vi "HV Onstate Multi.vi"(8 "On/Off":string[](array[string]), 11 "Channel":string[](array[string])) -> (3 "standard output":string)   [LabVIEW 2018, in "HV QMH.lvlib"]
uses:
  HV QMH.lvlib
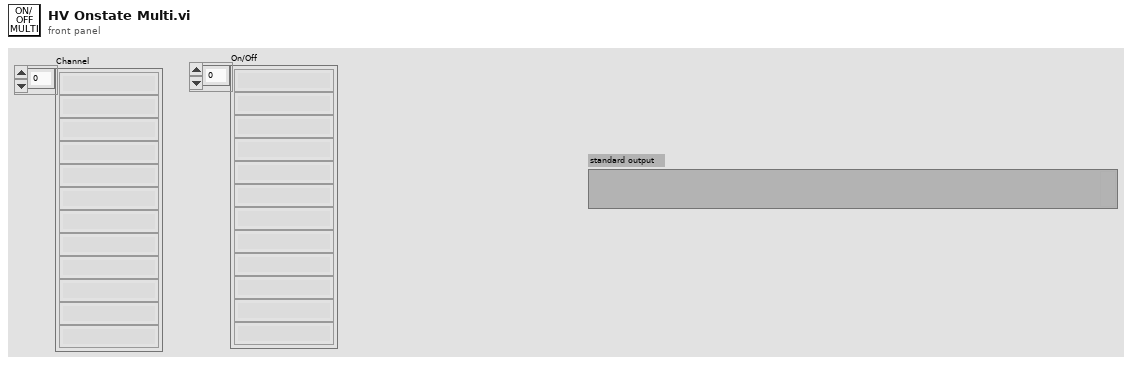
[diagram p1: front panel]
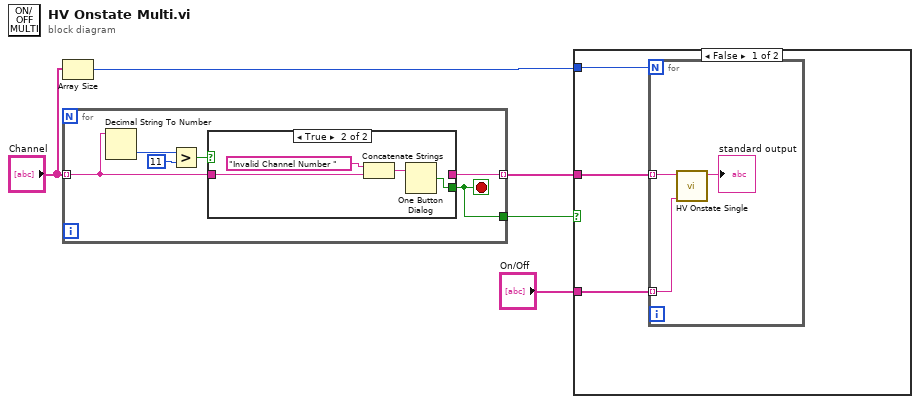
[diagram p0: block diagram]
diagram:
  n1 = Array Size(array="Channel") -> (size(s)=w5:i32)
  n2 = for {
    tunnel: "Channel" -> [w11] mode=indexing
    tunnel: [w10] -> w2 mode=indexing
    tunnel: [w6] -> w1
    stop <- w6 stop-if-true
    n3 = Decimal String To Number(string=w11) -> (number=w9:i32)  [unwired: 2 in, 1 out]
    n4 = Greater?(x=w9, y=11) -> (0:w8:bool)
    n5 = case shown="True" w8 {
      tunnel: w11 -> [w12 w13]
      tunnel: [w12 _] -> w10
      tunnel: [_ w16] -> w6
      frame False {
      }
      frame True {
        n6 = Concatenate Strings("Invalid Channel Number " ("message"), w13) -> (w14:string)
        n7 = One Button Dialog(message=w14) -> (true=w16:bool)  [unwired: 1 in]
      }
    }
  }
  n8 = case shown="False" w1 {
    tunnel: w5 -> [w19 _]
    tunnel: "On/Off" -> [w18 _]
    tunnel: w2 -> [w17 _]
    frame False {
      n9 = for {
        N: w19 -> [_]
        tunnel: w17 -> [w22] mode=indexing
        tunnel: w18 -> [w21] mode=indexing
        n10 = call "HV Onstate Single.vi"("On/Off"=w21, "Channel"=w22) -> ("standard output"=→"standard output":string)  [unwired: 9 in]
      }
    }
    frame True {
    }
  }
